vi "Read File.vi"(8 "error in (no error)":errorcluster, 11 "CSV File":path) -> (0 "error in (no error) 2":errorcluster, 2 "Data":string[][](array[string]))   [LabVIEW 2024]
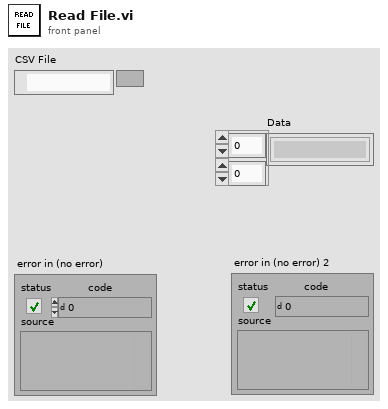
[diagram p1: front panel]
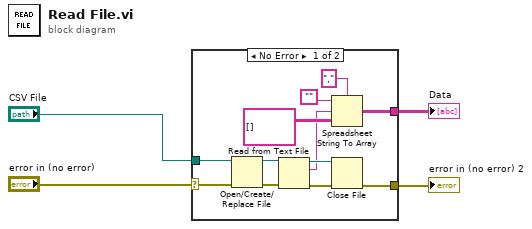
[diagram p0: block diagram]
diagram:
  n1 = case shown="No Error" "error in (no error)" {
    selector: "error in (no error)" -> [w16 w17]
    tunnel: "CSV File" -> [w11 _]
    tunnel: [w10 w17] -> w2
    tunnel: [w5 _] -> w1
    frame No Error {
      n2 = Open/Create/Replace File(file path (use dialog)=w11, error in=w16) -> (refnum out=w15:refnum<file>, error out=w14:errorcluster)  [unwired: 4 in, 1 out]
      n3 = Read from Text File(file (use dialog)=w15, error in=w14) -> (refnum out=w13:refnum<file>, text=w7:string, error out=w12:errorcluster)  [unwired: 2 in, 1 out]
      n4 = Spreadsheet String To Array(delimiter (Tab)=",", format string="", spreadsheet string=w7, array type (2D Dbl)=string[][] []) -> (array=w5:string[][])
      n5 = Close File(refnum=w13, error in=w12) -> (error out=w10:errorcluster)  [unwired: 1 out]
    }
    frame Error {
    }
  }
  "error in (no error) 2" <- w2
  "Data" <- w1
